vi "Last Frame.vi"(8 "error in (no error)":errorcluster, 11 "[V] Main UI in":refnum<class "[V] Main UI.lvclass">) -> (0 "error out":errorcluster, 3 "[V] Main UI out":refnum<class "[V] Main UI.lvclass">)   [LabVIEW 2020, in "[V] Main UI.lvlib" / "[V] Main UI.lvclass"]
uses:
  [V] Main UI.lvclass
  [V] Main UI.lvclass/[V] Main UI.ctl
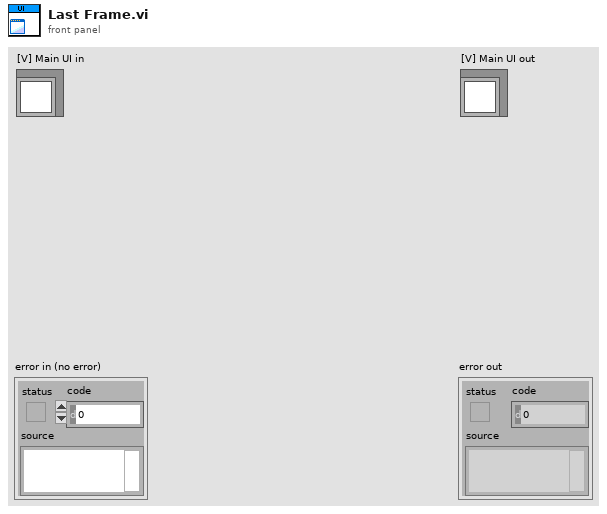
[diagram p1: front panel]
types:
  T1 = typedef "number.ctl" = i8
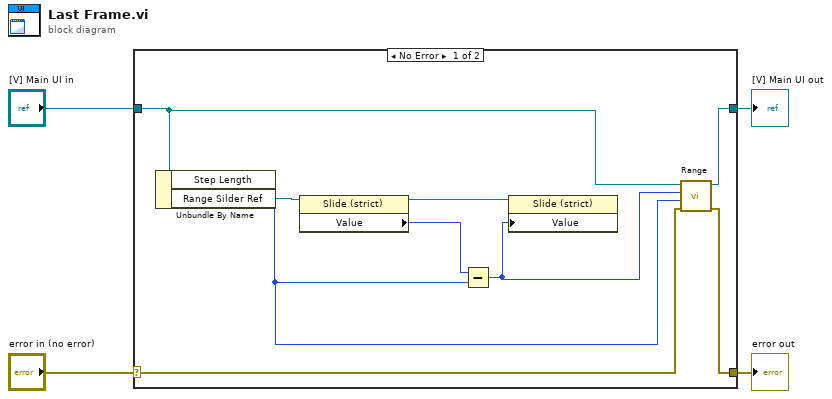
[diagram p0: block diagram]
diagram:
  n1 = case shown="No Error" "error in (no error)" {
    selector: "error in (no error)" -> [w6 w15]
    tunnel: [w5 w15] -> w3
    tunnel: [w10 w14] -> w1
    tunnel: "[V] Main UI in" -> [w11 w14]
    frame No Error {
      n2 = Unbundle By Name(w11) -> ("Step Length"=w7:u8, "Range Silder Ref"=w13:refnum<vi>)
      n3 = property class="Slide (strict)"(reference=w13) -> (reference out=w9:refnum<vi>, "Value"=w12:T1)  [unwired: 1 in, 1 out]
      n4 = Subtract(x=w12, y=w7) -> (x-y=w8:u8)
      n5 = property class="Slide (strict)"(reference=w9, "Value"=w8) -> ()  [unwired: 1 in, 2 out]
      n6 = call "Range.vi"("error in (no error)"=w6, "length"=w7, "index"=w8, "[V] Main UI in"=w11) -> ("error out"=w5:errorcluster, "[V] Main UI out"=w10:refnum<class "[V] Main UI.lvclass">)  [unwired: 6 in]
    }
    frame Error {
    }
  }
  "error out" <- w3
  "[V] Main UI out" <- w1
